vi "Mouse Up.vi"(8 "error in (no error)":errorcluster, 10 "Point":cluster{"x":i16, "y":i16}, 11 "Graphic in":refnum<class "Graphic.lvclass">) -> (0 "error out":errorcluster, 3 "Graphic out":refnum<class "Graphic.lvclass">)   [LabVIEW 2015, in "Graphic.lvclass"]
uses:
  Graphic.lvclass
  Graphic.lvclass/Graphic.ctl
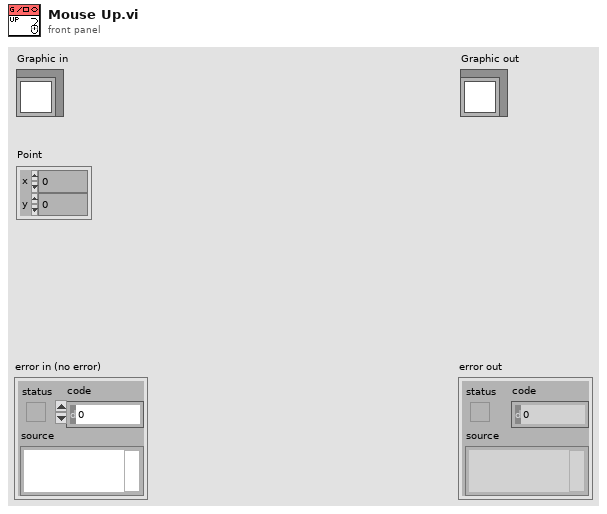
[diagram p1: front panel]
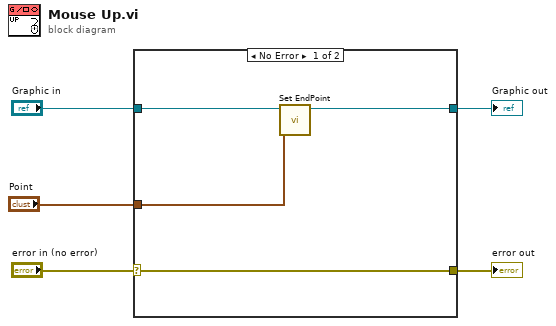
[diagram p0: block diagram]
diagram:
  n1 = case shown="No Error" "error in (no error)" {
    selector: "error in (no error)" -> [w8 w11]
    tunnel: [w8 w11] -> w4
    tunnel: [w7 w10] -> w2
    tunnel: "Graphic in" -> [w9 w10]
    tunnel: "Point" -> [w6 _]
    frame No Error {
      n2 = call "Set EndPoint.vi"("EndPoint"=w6, "Graphic in"=w9) -> ("Graphic out"=w7:refnum<class "Graphic.lvclass">)  [unwired: 8 in, 1 out]
    }
    frame Error {
    }
  }
  "error out" <- w4
  "Graphic out" <- w2
